vi "OSICS_Read_Status_Byte.vi"(8 "error in":errorcluster, 11 "VISA IN":refnum<visa-resource-name>) -> (0 "error out":errorcluster, 2 "SBR":bool[](array[boolean]) caption="Array", 3 "VISA OUT":refnum<visa-resource-name>)   [LabVIEW 2014, in "OSICS_LIB.lvlib"]
doc: "Decodes the status byte register into an array of boolean.\nBit7 : OPC condition\nBit5 : ESB Condition\nBit4 : MAV condition \n\nGPIB only"
uses:
  OSICS_LIB.lvlib
panel:
  # "0"
  # "1"
  # "2"
  # "..."
  # "7"
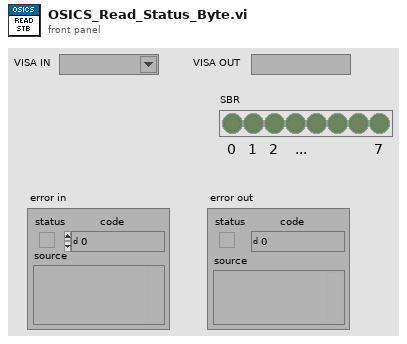
[diagram p1: front panel]
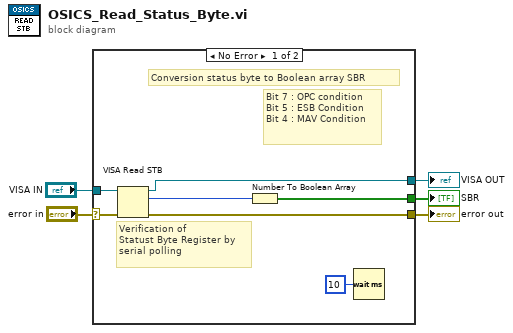
[diagram p0: block diagram]
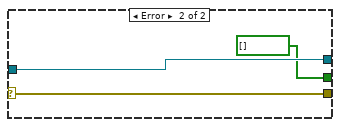
[diagram p2: hidden frame]
diagram:
  n1 = case shown="No Error" "error in" {
    selector: "error in" -> [w7 w14]
    tunnel: [w12 bool[] [] ("Boolean array")] -> w5
    tunnel: "VISA IN" -> [w10 w15]
    tunnel: [w9 w15] -> w3
    tunnel: [w8 w14] -> w2
    frame No Error {
      # "Verification of \nStatust Byte Register by\nserial polling"
      # "Bit 7 : OPC condition\nBit 5 : ESB Condition\nBit 4 : MAV Condition"
      # "Conversion status byte to Boolean array SBR"
      n2 = VISA Read STB(8:w7, 11:w10) -> (0:w8:errorcluster, 2:w11:u16, 3:w9:refnum<visa-resource-name>)
      n3 = Number To Boolean Array(number=w11) -> (Boolean array=w12:bool[])
      n4 = Wait (ms)(milliseconds to wait=u32 10) -> ()  [unwired: 1 out]
    }
    frame Error {
    }
  }
  "SBR" <- w5
  "error out" <- w2
  "VISA OUT" <- w3
